vi "Harness source and built code.vi"(8 "error in (no error)":errorcluster, 10 "Action":string, 11 "Class":path=path "C:/git/labview-icon-editor/Sandbox/Class 2/_Class.lvclass") -> (0 "error out":errorcluster)   [LabVIEW 2021]
uses:
  <resource>/plugins/IconEditorInterface.lvlibp/HarnessInterface/IconEditorInterface.lvclass
  HarnessInterface/_IconEditorInterface.lvclass
panel:
  # "C:\\git\\labview-icon-editor\\builds\\Sandbox\\Class Harness\\Class.lvlibp\\Class 2\\Class.lvclass"
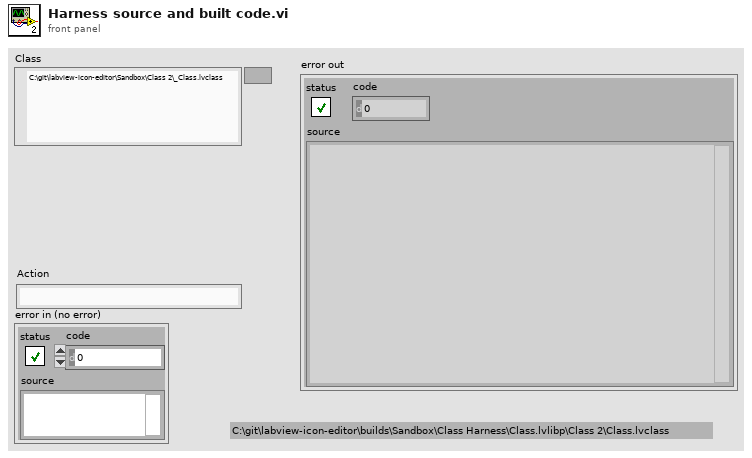
[diagram p1: front panel]
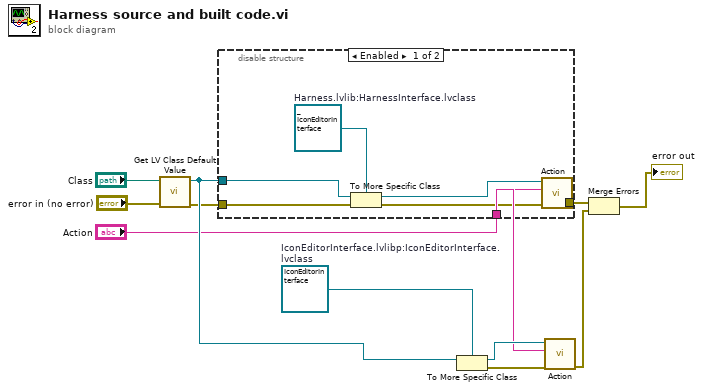
[diagram p0: block diagram]
diagram:
  w7 = refnum<class "IconEditorInterface.lvclass"> refnum  # IconEditorInterface.lvlibp:IconEditorInterface.lvclass
  n1 = call <vilib>:"Get LV Class Default Value.vi"("error in (no error)"="error in (no error)", "class path"="Class") -> ("error out"=w8:errorcluster, "object"=w9:refnum<class>)  [unwired: 8 in]
  n2 = disable-structure shown="Enabled" {
    disable-tunnel: w9 -> [w16 _]
    disable-tunnel: w8 -> [w15 _]
    disable-tunnel: "Action" -> [w14 _]
    disable-tunnel: [w13 _] -> w3
    frame Enabled {
      w18 = refnum<class "_IconEditorInterface.lvclass"> refnum  # Harness.lvlib:HarnessInterface.lvclass
      n3 = To More Specific Class(target class=w18, reference=w16, error in=w15) -> (specific class reference=w17:refnum<class "_IconEditorInterface.lvclass">, error out=w12:errorcluster)
      n4 = call-dynamic "Action.vi"("error in (no error)"=w12, "Action"=w14, "HarnessInterface in"=w17) -> ("error out"=w13:errorcluster)  [unwired: 7 in, 1 out]
    }
    frame Disabled {
    }
  }
  n5 = To More Specific Class(target class=w7, reference=w9) -> (specific class reference=w5:refnum<class "IconEditorInterface.lvclass">, error out=w6:errorcluster)  [unwired: 1 in]
  n6 = call-dynamic "Action.vi"("error in (no error)"=w6, "Action"="Action", "HarnessInterface in"=w5) -> ("error out"=w2:errorcluster)  [unwired: 7 in, 1 out]
  n7 = Merge Errors(w3, w2) -> (→"error out":errorcluster)
